vi "CONF device create digital.vi"(7 "Config Digital Channels":T1, 10 "device in":tag) -> (1 "Sen":tag, 2 "Sdata":tag, 3 "Scl":tag)   [LabVIEW 2014]
uses:
  Kontrolki/KartaDAQ/CONF digital channel config.ctl
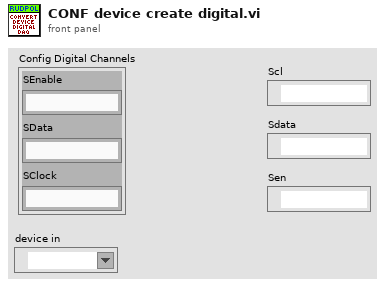
[diagram p1: front panel]
types:
  T1 = typedef "CONF digital channel config.ctl" = cluster{"SEnable":string, "SData":string, "SClock":string}
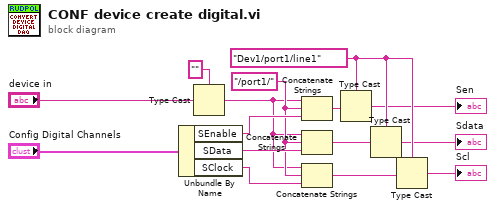
[diagram p0: block diagram]
diagram:
  w15 = tag "Dev1/port1/line1" ("lines")
  w9 = "/port1/" ("element")
  n1 = Unbundle By Name("Config Digital Channels") -> ("SEnable"=w12:string, "SData"=w10:string, "SClock"=w11:string)
  n2 = Type Cast(type="", x="device in") -> (*(type *) &x=w8:string)
  n3 = Concatenate Strings(w8, w9, w12) -> (w7:string)
  n4 = Concatenate Strings(w8, w9, w10) -> (w13:string)
  n5 = Concatenate Strings(w8, w9, w11) -> (w14:string)
  n6 = Type Cast(type=w15, x=w7) -> (*(type *) &x=→"Sen":tag)
  n7 = Type Cast(type=w15, x=w13) -> (*(type *) &x=→"Sdata":tag)
  n8 = Type Cast(type=w15, x=w14) -> (*(type *) &x=→"Scl":tag)
